vi "Read Engine State.vi"(0 "class data in":refnum<class "MB_ENGINE.lvclass">, 11 "error in (no error)":errorcluster) -> (4 "class data out":refnum<class "MB_ENGINE.lvclass">, 6 "Engine State":T1 items=["ACCELERATING", "DECELERATINGTOSTOP", "DECELERATING", "STEADY", "INDEX_ACCEL", "NDEX_RUN", "INDEX_DECEL", "INDEX_DWELL", "INACTIVE", "STANDBY", "STANDBYTOINACTIVE"], 15 "error out":errorcluster)   [LabVIEW 2019, in "MB_ENGINE.lvclass"]
uses:
  MB_ENGINE.lvclass
  Engine State.ctl
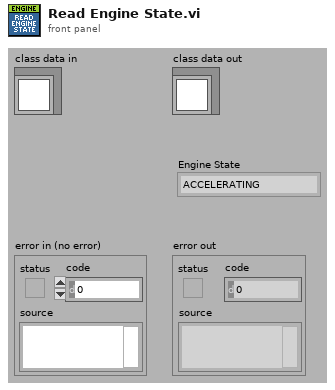
[diagram p1: front panel]
types:
  T1 = typedef "MB_ENGINE.lvclass/Engine State.ctl" = u16
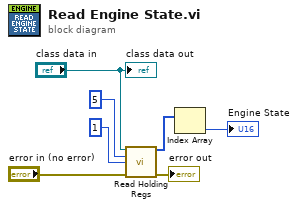
[diagram p0: block diagram]
diagram:
  n1 = call-dynamic "Read Holding Regs.vi"("reference in"="class data in", "starting address"=u16 5, "number of inputs"=u16 1, "error in (no error)"="error in (no error)") -> ("register values"=w1:u16[], "error out"=→"error out":errorcluster)  [unwired: 10 in]
  n2 = Index Array(array=w1) -> (element=→"Engine State":u16)  [unwired: 1 in]
  "class data out" <- "class data in"
